vi "ScanForBricks.vi"(8 "error in (no error)":errorcluster, 10 "Scan Wireless":bool, 11 "VIAManager in":refnum<class "VIAManager.lvclass">) -> (0 "error out":errorcluster, 3 "VIAManager out":refnum<class "VIAManager.lvclass">)   [LabVIEW 2012, in "VIAManager.lvclass"]
uses:
  <vilib>/NXT/LegoClasses/BrickManagers/VIAManager/VIAManager.lvclass
  <vilib>/NXT/LegoClasses/BrickManagers/VIAManager/VIAManager.lvclass/VIAManager.ctl
  <vilib>/NXT/LegoClasses/BrickManagers/Base/BrickManager.lvclass
  <vilib>/NXT/LegoClasses/VIA/VIA.lvclass
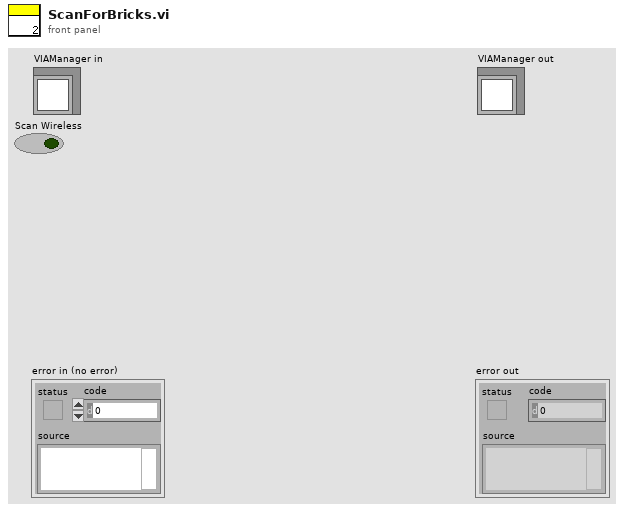
[diagram p1: front panel]
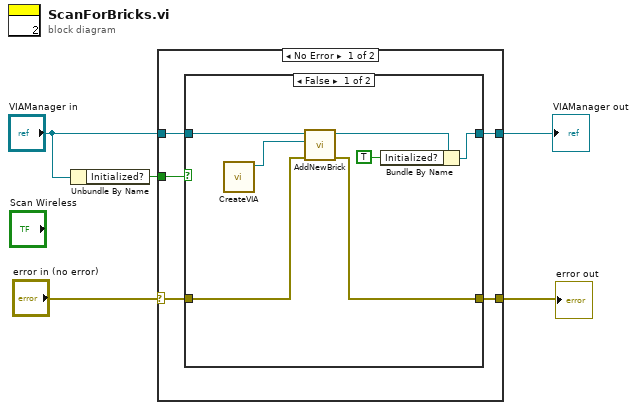
[diagram p0: block diagram]
diagram:
  n1 = Unbundle By Name("VIAManager in") -> ("Initialized?"=w4:bool)
  n2 = case shown="No Error" "error in (no error)" {
    selector: "error in (no error)" -> [w7 w20]
    tunnel: w4 -> [w10 _]
    tunnel: "VIAManager in" -> [w9 w21]
    tunnel: [w8 w21] -> w2
    tunnel: [w6 w20] -> w1
    frame No Error {
      n3 = case shown="False" w10 {
        tunnel: w9 -> [w17 w19]
        tunnel: [w15 w19] -> w8
        tunnel: w7 -> [w14 w18]
        tunnel: [w13 w18] -> w6
        frame False {
          n4 = call <vilib>:"CreateVIA.vi"() -> ("VIA.lvclass"=w11:refnum<class "VIA.lvclass">)  [unwired: 11 in]
          n5 = call <vilib>:"AddNewBrick.vi"("error in (no error)"=w14, "Brick"=w11, "BrickManager in"=w17) -> ("error out"=w13:errorcluster, "BrickManager out"=w16:refnum<class "VIAManager.lvclass">)  [unwired: 7 in]
          n6 = Bundle By Name(cluster=w16, "Initialized?"=TRUE) -> (w15:refnum<class "VIAManager.lvclass">)
        }
        frame True {
        }
      }
    }
    frame Error {
    }
  }
  "error out" <- w1
  "VIAManager out" <- w2
